vi "getWavelength_v80AM9.vi"() -> ()   [LabVIEW 2016]
uses:
  <vilib>/Analysis/NI_AALBase.lvlib
  <vilib>/Analysis/baseanly.llb/Mean (DBL).vi
  x32/CLDevIFace.dll
panel:
  out "NewFilePath":path
  out "NewFileCreated":string
  in  "ProjectName":string="QFinger"
  in  "Folder path input":path=path "C:/Labview34970A stuff/Data"
  out "Wavelength":dbl format="%0.5f"
  out "0.75ppm in Wave (nm)":dbl format="%#_3g"
  out "0.75ppm in Freq (MHz)":dbl
  out "Freq (Hz)":dbl
  out "standard dev":dbl format="%0.5f"
  in  "# for Stdev":i32=7
  in  "Avg":i32=1
  out "Delta MHz":dbl
  in  "Scale Factor":dbl=800.0
  out "Power (mW)":dbl format="%.9f"
  in  "Clear Chart?":bool
  in  "Delay Time (s)":dbl=0.01
  out "Wavelength vs time":cluster{dbl[], dbl[]}(graph)
  out "error out":errorcluster
  out "output param":i32
  in  "stop":bool
  in  "OK Button":bool
  in  "CommPort":dbl=5.0 caption="Comm Port #"
  # "Pr = 605.977 nm"
  # "Super cavity FSR  6 GHz\nZerodure FSR  750 MHz"
  # "1 pm = 200 MHz @1212nm\n1 pm = 800 MHz @606 nm"
  # "Bristol 621B accuracy = 0.75 ppm\nuseful conversions:"
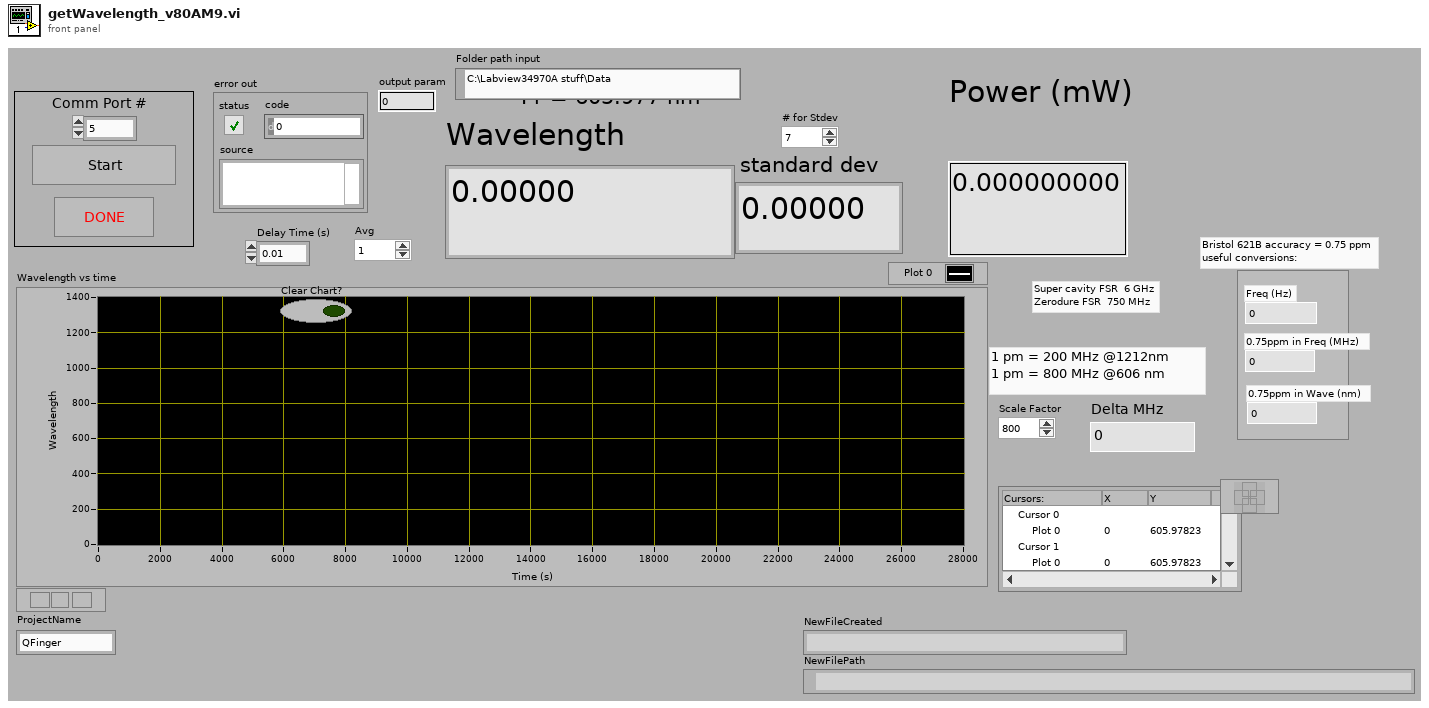
[diagram p1: front panel]
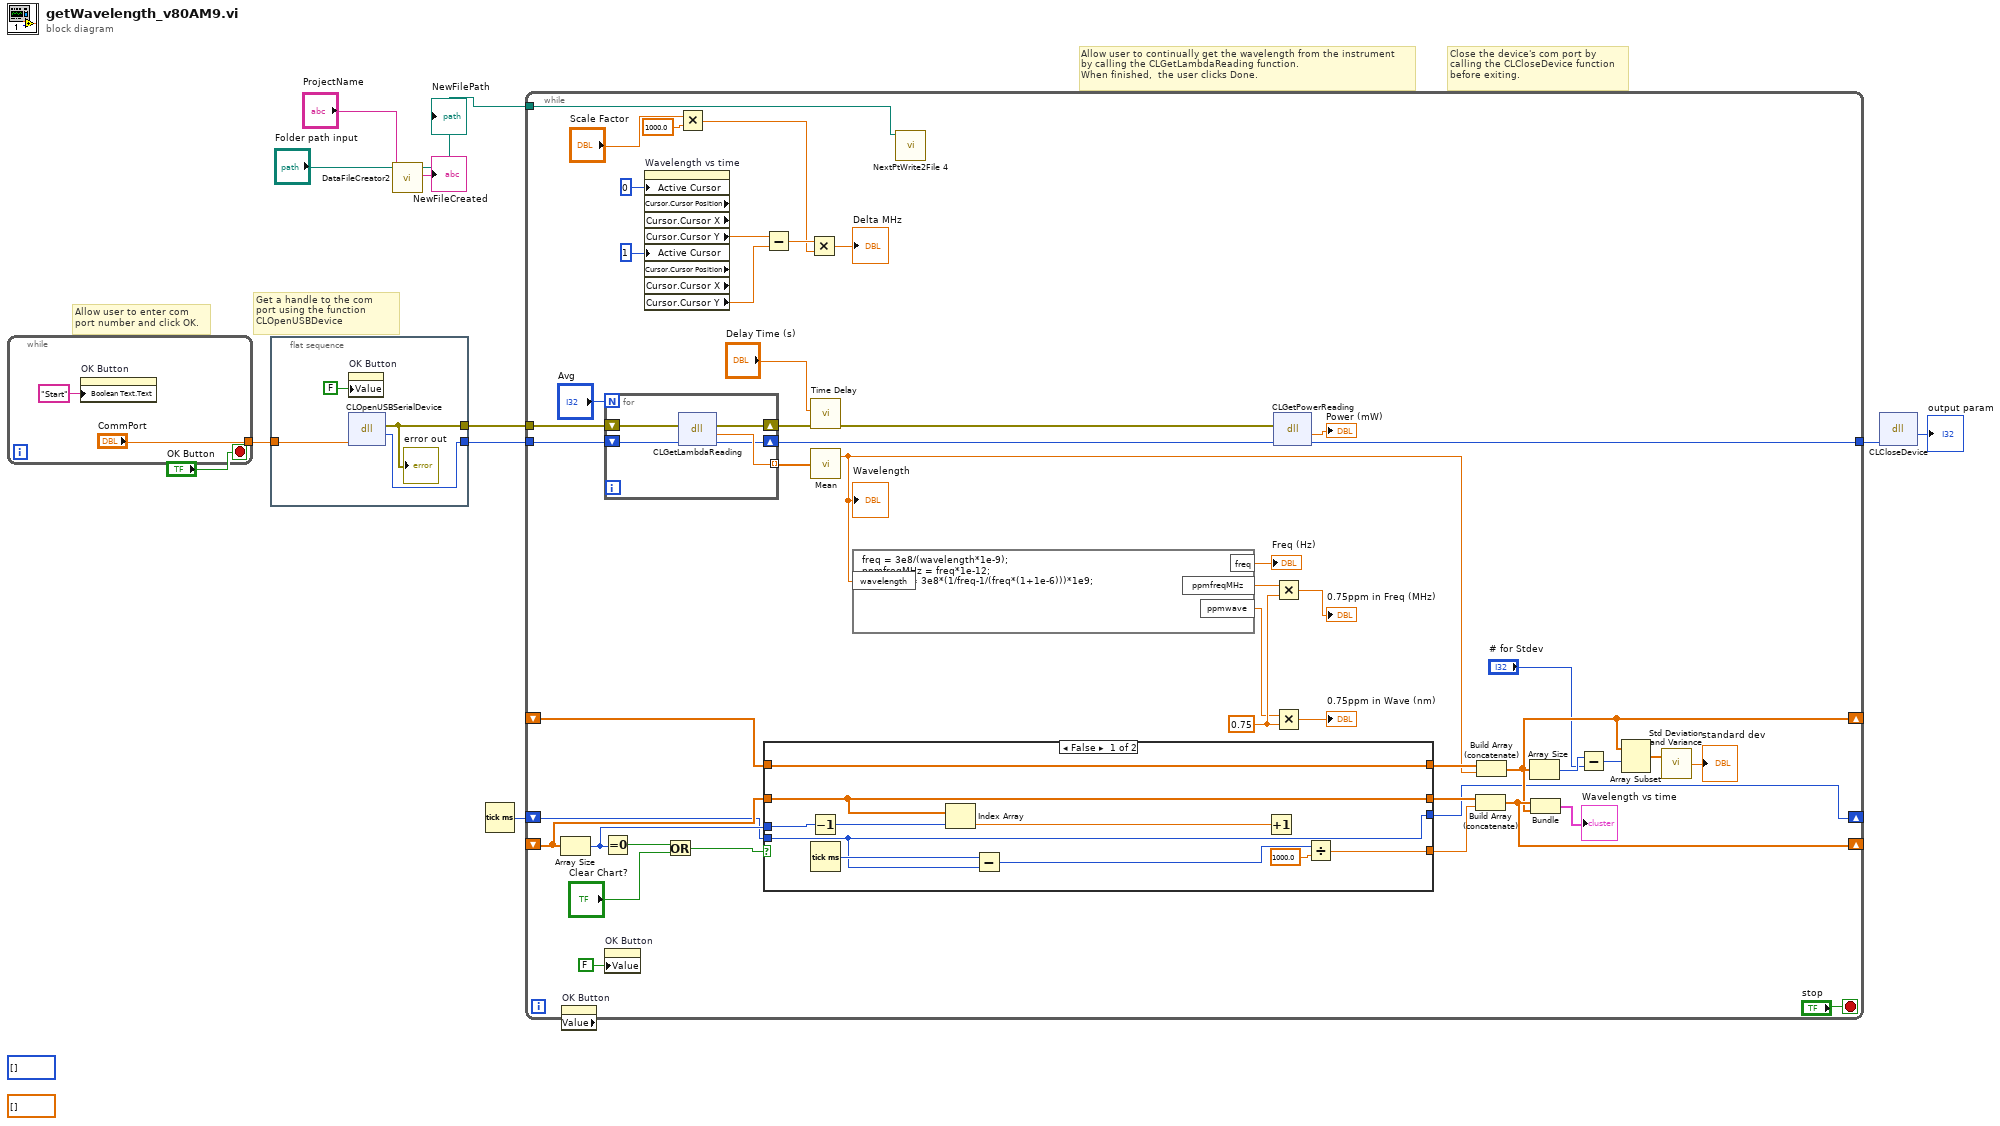
[diagram p0: block diagram]
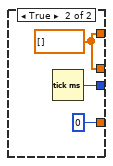
[diagram p2: hidden frame]
diagram:
  (unwired) i32[] []
  (unwired) dbl[] []
  # "Close the device's com port by\ncalling the CLCloseDevice function\nbefore exiting."
  # "Allow user to continually get the wavelength from the instrument\nby calling the CLGetLambdaReading function.  \nWhen finished,  the user clicks Done."
  # "Get a handle to the com\nport using the function CLOpenUSBDevice"
  # "Allow user to enter com \nport number and click OK."
  n1 = while {
    tunnel: ["CommPort"] -> w10
    stop <- "OK Button" stop-if-true
    n2 = property on="OK Button" class="Bool (strict)"("Boolean Text.Text"="Start") -> ()  [unwired: 2 in, 2 out]
  }
  n3 = flat-sequence {
    tunnel: w10 -> [w17]
    tunnel: [w16] -> w9
    tunnel: [w14] -> w6
    frame #0 {
      n4 = property on="OK Button" class="Bool (strict)"("Value"=FALSE) -> ()  [unwired: 2 in, 2 out]
      n5 = dll-call lib="C:/Users/Lab/Desktop/Bristol wavemeter 621/00424-2-00 621 customer CD/Programming Interface/x32/CLDevIFace.dll" fn="CLOpenUSBSerialDevice"("commPort"=w17) -> (error out=w14:errorcluster, "return type"=w16:i32)  [unwired: 4 in, 1 out]
      "error out" <- w14
    }
  }
  n6 = call "DataFileCreator2.vi"("ProjectName"="ProjectName", "Folder path input"="Folder path input") -> ("NewFileCreated"=→"NewFileCreated":string, "NewFilePath"=w1:path)  [unwired: 8 in]
  "NewFilePath" <- w1
  n7 = Tick Count (ms)() -> (millisecond timer value=w5:u32)
  n8 = while {
    tunnel: w9 -> [w65]
    tunnel: [w53] -> w8
    shift-right: [w33] -> _
    shift-left: _ -> [w57]
    shift-right: [w62] -> _
    shift-left: _ -> [w38]
    tunnel: w6 -> [w58]
    shift-right: [w19] -> _
    shift-left: w5 -> [w20]
    tunnel: w1 -> [w18]
    stop <- "stop" stop-if-true
    w23 = 0.75 ("y")
    n9 = Array Size(array=w38) -> (size(s)=w35:i32)
    n10 = property on="OK Button" class="Bool (strict)" props=["Value"]() -> ()  [unwired: 2 in, 3 out]
    n11 = Equal To 0?(x=w35) -> (x = 0?=w43:bool)
    n12 = for {
      N: "Avg" -> [_]
      tunnel: [w69] -> w36 mode=indexing
      shift-right: [w66] -> w54
      shift-left: w65 -> [w70]
      shift-right: [w68] -> w59
      shift-left: w58 -> [w67]
      n13 = dll-call lib="C:/Users/Lab/Desktop/Bristol wavemeter 621/00424-2-00 621 customer CD/Programming Interface/x32/CLDevIFace.dll" fn="CLGetLambdaReading"(error in=w67, "devHandle"=w70) -> (error out=w68:errorcluster, "return type"=w69:dbl, "devHandle"=w66:i32)  [unwired: 2 in, 1 out]
    }
    n14 = property on="OK Button" class="Bool (strict)"("Value"=FALSE) -> ()  [unwired: 2 in, 2 out]
    n15 = property on="Wavelength vs time" class="XYGraph (strict)" props=["Active Cursor", "Cursor", "Cursor Position", "Cursor", "Cursor X", "Cursor", "Cursor Y", "Active Cursor", "Cursor", "Cursor Position", "Cursor", "Cursor X", "Cursor", "Cursor Y"]("Active Cursor"=u32 0, "Active Cursor"=u32 1) -> ("Cursor.Cursor Y"=w49:dbl, "Cursor.Cursor Y"=w50:dbl)  [unwired: 2 in, 6 out]
    n16 = Or(x=w43, y="Clear Chart?") -> (x .or. y?=w41:bool)
    n17 = Multiply(x="Scale Factor", y=1000.0) -> (x*y=w44:dbl)
    n18 = Subtract(x=w49, y=w50) -> (x-y=w51:dbl)
    n19 = case shown="False" w41 {
      tunnel: w57 -> [w80 _]
      tunnel: w38 -> [w79 _]
      tunnel: [w79 w81] -> w39
      tunnel: [w80 w81] -> w40
      tunnel: w35 -> [w77 _]
      tunnel: [w72 0] -> w34
      tunnel: w20 -> [w71 _]
      tunnel: [w71 w82] -> w19
      frame False {
        n20 = Decrement(x=w77) -> (x-1=w76:i32)
        n21 = Tick Count (ms)() -> (millisecond timer value=w75:u32)
        n22 = Index Array(array=w79, index=w76) -> (element=w78:dbl)
        n23 = Subtract(x=w75, y=w71) -> (x-y=w73:u32)
        n24 = Increment(x=w78) -> ()  [unwired: 1 out]
        n25 = Divide(x=w73, y=1000.0) -> (x/y=w72:dbl)
      }
      frame True {
        w81 = dbl[] []
        n26 = Tick Count (ms)() -> (millisecond timer value=w82:u32)
      }
    }
    n27 = Multiply(x=w51, y=w44) -> (x*y=→"Delta MHz":dbl)
    n28 = call "Time Delay"("error in (no error)"=w59, "Delay Time (s)"="Delay Time (s)") -> ("error out"=w56:errorcluster)  [unwired: 9 in]
    n29 = call-poly <vilib>:"Mean.vi"("X"=w36) -> ("mean"=w26:dbl)  [unwired: 1 out]
    "Wavelength" <- w26
    n30 = formula code="freq = 3e8/(wavelength*1e-9);\nppmfreqMHz = freq*1e-12;\nppmwave = 3e8*(1/freq-1/(freq*(1+1e-6)))*1e9;"("wavelength"=w26) -> ("freq"=→"Freq (Hz)":dbl, "ppmfreqMHz"=w25:dbl, "ppmwave"=w22:dbl)
    n31 = call "NextPtWrite2File 4.vi"("Folder path input"=w18) -> ()  [unwired: 9 in, 2 out]
    n32 = dll-call lib="C:/Users/Lab/Desktop/Bristol wavemeter 621/00424-2-00 621 customer CD/Programming Interface/x32/CLDevIFace.dll" fn="CLGetPowerReading"(error in=w56, "devHandle"=w54) -> ("return type"=→"Power (mW)":dbl, "devHandle"=w53:i32)  [unwired: 2 in, 2 out]
    n33 = Multiply(x=w25, y=w23) -> (x*y=→"0.75ppm in Freq (MHz)":dbl)
    n34 = Multiply(x=w22, y=w23) -> (x*y=→"0.75ppm in Wave (nm)":dbl)
    n35 = Build Array (concatenate)(w39, w34) -> (w62:dbl[])
    n36 = Build Array (concatenate)(w40, w26) -> (w33:dbl[])
    n37 = Array Size(array=w33) -> (size(s)=w32:i32)
    n38 = Bundle(w62, w33) -> (→"Wavelength vs time":cluster{dbl[], dbl[]})  [unwired: 1 in]
    n39 = Subtract(x=w32, y="# for Stdev") -> (x-y=w30:i32)
    n40 = Array Subset(array=w33, index=w30) -> (w29:dbl[])  [unwired: 1 in]
    n41 = call <vilib>:"Std Deviation and Variance.vi"("X"=w29) -> ("standard deviation"=→"standard dev":dbl)  [unwired: 1 in, 2 out]
  }
  n42 = dll-call lib="C:/Users/Lab/Desktop/Bristol wavemeter 621/00424-2-00 621 customer CD/Programming Interface/x32/CLDevIFace.dll" fn="CLCloseDevice"("commPort"=w8) -> ("return type"=→"output param":i32)  [unwired: 4 in, 2 out]
